vi "Resize CaseStructure By Making Space.vi"(8 "error in (no error)":errorcluster, 10 "Bounds":T1, 11 "CSM-Helper in":refnum<class "CSM-Helper.lvclass">) -> (0 "error out":errorcluster, 1 "DiffBound":T1, 2 "MakeSpace.Rect":T2, 3 "CSM-Helper out":refnum<class "CSM-Helper.lvclass">)   [LabVIEW 2020, in "CSM-Helper.lvclass"]
uses:
  CSM-Helper.lvclass
  <vilib>/Utility/miscctls.llb/LVBoundsTypeDef.ctl
  <vilib>/Utility/miscctls.llb/LVRectTypeDef.ctl
  CSM-Helper.lvclass/CSM-Helper.ctl
  Properties/Read Back Tunnels Refs.vi
  Properties/Read Case Structure Ref.vi
  Properties/Read Block Diagram Ref.vi
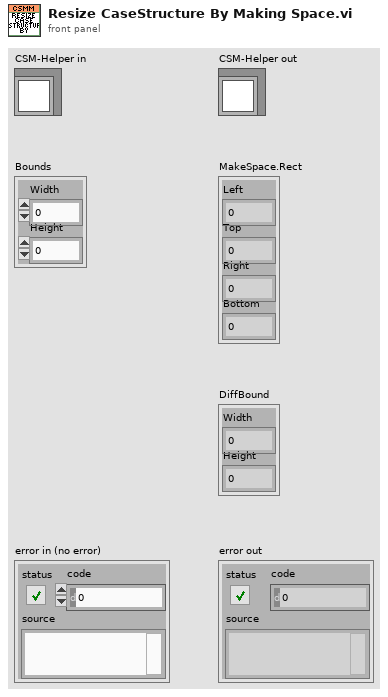
[diagram p1: front panel]
types:
  T1 = typedef "LVBoundsTypeDef.ctl" = cluster{"Width":u32, "Height":u32}
  T2 = typedef "LVRectTypeDef.ctl" = cluster{"Left":i16, "Top":i16, "Right":i16, "Bottom":i16}
  T3 = typedef "CSM-Helper.lvclass/_csmhelper_Back_Tunnels_Refs.ctl" = cluster{"InternalData":refnum<vi>, "Resp":refnum<vi>, "Remaining State":refnum<vi>, "Error":refnum<vi>}
  T4 = typedef "LVPositionTypeDef.ctl" = cluster{"Left":i32, "Top":i32}
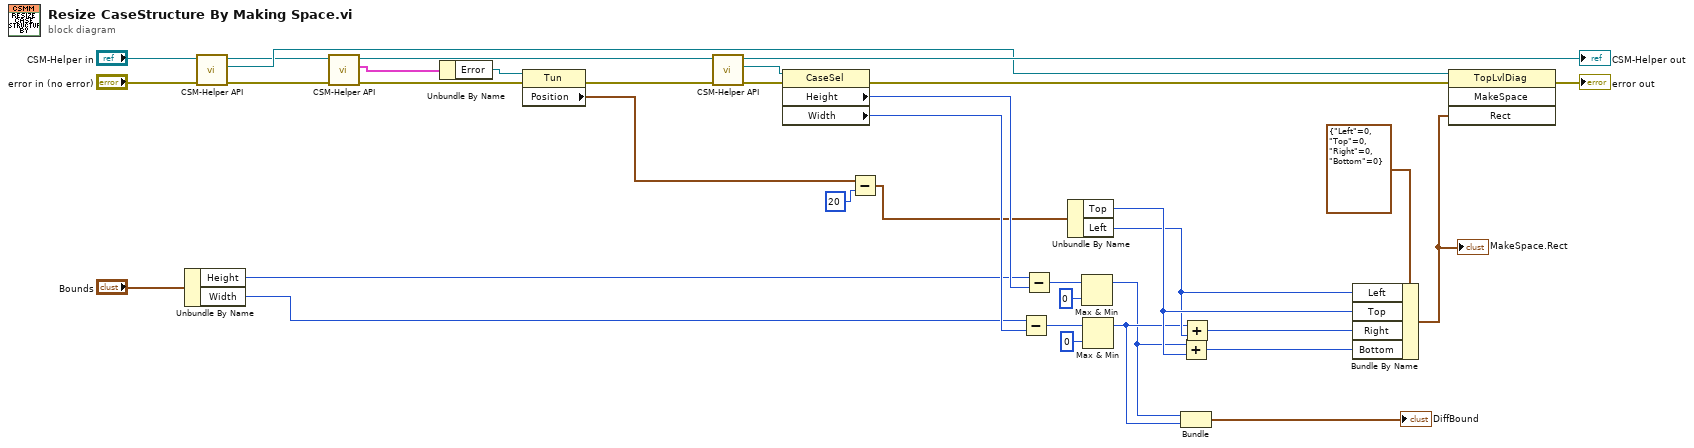
[diagram p0: block diagram]
diagram:
  n1 = Unbundle By Name("Bounds") -> ("Height"=w16:u32, "Width"=w17:u32)
  n2 = call-poly "CSM-Helper API.vi"("error in (no error)"="error in (no error)", "CSM-Helper in"="CSM-Helper in") -> ("error out"=w10:errorcluster, "Diagram"=w32:refnum<vi>, "CSM-Helper out"=w9:refnum<class "CSM-Helper.lvclass">)  [unwired: 7 in]
  n3 = call-poly "CSM-Helper API.vi"("error in (no error)"=w10, "CSM-Helper in"=w9) -> ("error out"=w8:errorcluster, "Back Tunnels"=w5:T3, "CSM-Helper out"=w7:refnum<class "CSM-Helper.lvclass">)  [unwired: 7 in]
  n4 = Unbundle By Name(w5) -> ("Error"=w4:refnum<vi>)
  n5 = property class="Tun"(reference=w4, error in=w8) -> (error out=w6:errorcluster, "Position"=w3:T4)  [unwired: 1 out]
  n6 = call-poly "CSM-Helper API.vi"("error in (no error)"=w6, "CSM-Helper in"=w7) -> ("error out"=w28:errorcluster, "Case Structure"=w29:refnum<vi>, "CSM-Helper out"=→"CSM-Helper out":refnum<class "CSM-Helper.lvclass">)  [unwired: 7 in]
  n7 = property on="Property Node" class="CaseSel"(reference=w29, error in=w28) -> (error out=w27:errorcluster, "Height"=w26:u32, "Width"=w25:u32)  [unwired: 1 out]
  n8 = Subtract(x=w3, y=u32 20 ("Height")) -> (x-y=w1:cluster{"Left":u32, "Top":u32})
  n9 = Subtract(x=w17, y=w25) -> (x-y=w23:u32)
  n10 = Subtract(x=w16, y=w26) -> (x-y=w20:u32)
  n11 = Unbundle By Name(w1) -> ("Top"=w15:u32, "Left"=w14:u32)
  n12 = Max & Min(x=w20, y=u32 0) -> (max(x,y)=w12:u32)  [unwired: 1 out]
  n13 = Max & Min(x=w23, y=u32 0) -> (max(x,y)=w13:u32)  [unwired: 1 out]
  n14 = Add(x=w12, y=w15) -> (x+y=w30:u32)
  n15 = Bundle(w12, w13) -> (→"DiffBound":cluster{u32, u32})  [unwired: 1 in]
  n16 = Add(x=w13, y=w14) -> (x+y=w31:u32)
  n17 = Bundle By Name(cluster=T2 {"Left"=0, "Top"=0, "Right"=0, "Bottom"=0} ("Rect"), "Left"=w14, "Top"=w15, "Right"=w31, "Bottom"=w30) -> (w24:T2)
  "MakeSpace.Rect" <- w24
  n18 = invoke on="Invoke Node" class="TopLvlDiag" method="MakeSpace"(reference=w32, error in=w27, "Rect"=w24) -> (error out=→"error out":errorcluster)  [unwired: 1 in, 3 out]
